vi "PM-GUI-add_visual_peak_detector.vi"(7 "Peak Detection":bool, 9 "Bottom":dbl, 10 "Top":dbl, 11 "waveform in":waveform(dbl)) -> (3 "Waveforms out":waveform(dbl)[](array[waveform]))   [LabVIEW 2020]
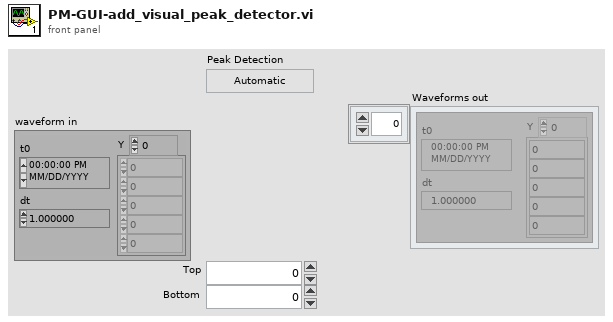
[diagram p1: front panel]
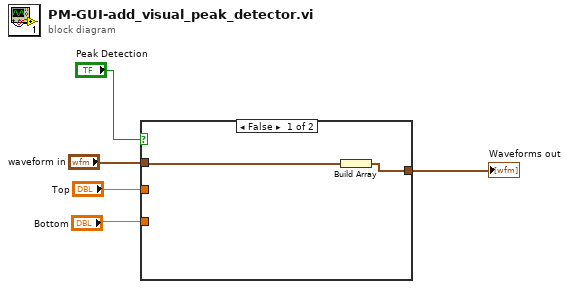
[diagram p0: block diagram]
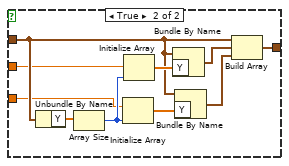
[diagram p2: hidden frame]
diagram:
  n1 = case shown="False" "Peak Detection" {
    tunnel: "waveform in" -> [w7 w11]
    tunnel: [w6 w10] -> w4
    tunnel: "Top" -> [_ w9]
    tunnel: "Bottom" -> [_ w8]
    frame False {
      n2 = Build Array(w7) -> (w6:waveform(dbl)[])
    }
    frame True {
      n3 = Unbundle By Name(w11) -> ("Y"=w17:dbl[])
      n4 = Array Size(array=w17) -> (size(s)=w16:i32)
      n5 = Initialize Array(w8, w16) -> (w15:dbl[])
      n6 = Initialize Array(w9, w16) -> (w14:dbl[])
      n7 = Bundle By Name(cluster=w11, "Y"=w14) -> (w12:waveform(dbl))
      n8 = Bundle By Name(cluster=w11, "Y"=w15) -> (w13:waveform(dbl))
      n9 = Build Array(w11, w12, w13) -> (w10:waveform(dbl)[])
    }
  }
  "Waveforms out" <- w4
